vi "Douglas_22082017.vi"() -> ()   [LabVIEW 2017]
uses:
  <vilib>/Utility/error.llb/DialogType.ctl
  <vilib>/DAQmx/read.llb/DAQmx Read (Analog 1D Wfm NChan NSamp).vi
  <vilib>/Analysis/baseanly.llb/Mean (DBL).vi
  <vilib>/Analysis/5stat.llb/RMS (DBL).vi
  Instance           1 15Saved   Douglas .vi
  <vilib>/Waveform/WDTFileIO.llb/Export Waveforms To Spreadsheet File (1D).vi
  <vilib>/DAQmx/create/channels.llb/DAQmx Create Channel (AI-Voltage-Basic).vi
  <vilib>/DAQmx/configure/timing.llb/DAQmx Timing (Sample Clock).vi
  <vilib>/DAQmx/miscellaneous.llb/DAQmx Fill In Error Info.vi
  <vilib>/Waveform/WDTFileIO.llb/ Write Waveforms to File (1D).vi
  <vilib>/Analysis/NI_AALBase.lvlib
  <vilib>/Analysis/NI_AALPro.lvlib
panel:
  in  "Pasta":path=path "D:/Box Sync/Doctoring/Testes/DEF"
  in  "Nome do Arquivo":string="CTL_usado_BBA-CC-1,20_pre7"
  in  "Aquisição C/T":bool=TRUE
  in  "Aqusiçao de Temperatura":bool=TRUE
  in  "Tempo Temperatura [s]":i32=3
  out "Temperature":dynamicdata(graph)
  out "Potencia Media":dbl format="%0.2f"
  out "Current/Voltage":waveform(dbl)[](graph)
  out "Tensão RMS":dbl format="%0.2f"
  out "Tensão Média":dbl format="%0.2f"
  out "Corrente RMS":dbl format="%0.2f"
  out "Corrente Média":dbl format="%0.2f"
  in  "Taxa de Aquisição":dbl=6000.0 format="%0.2f"
  in  "Tempo de C/T [s]":i32=3
  in  "Canal":tag="Dev1/ai0:1"
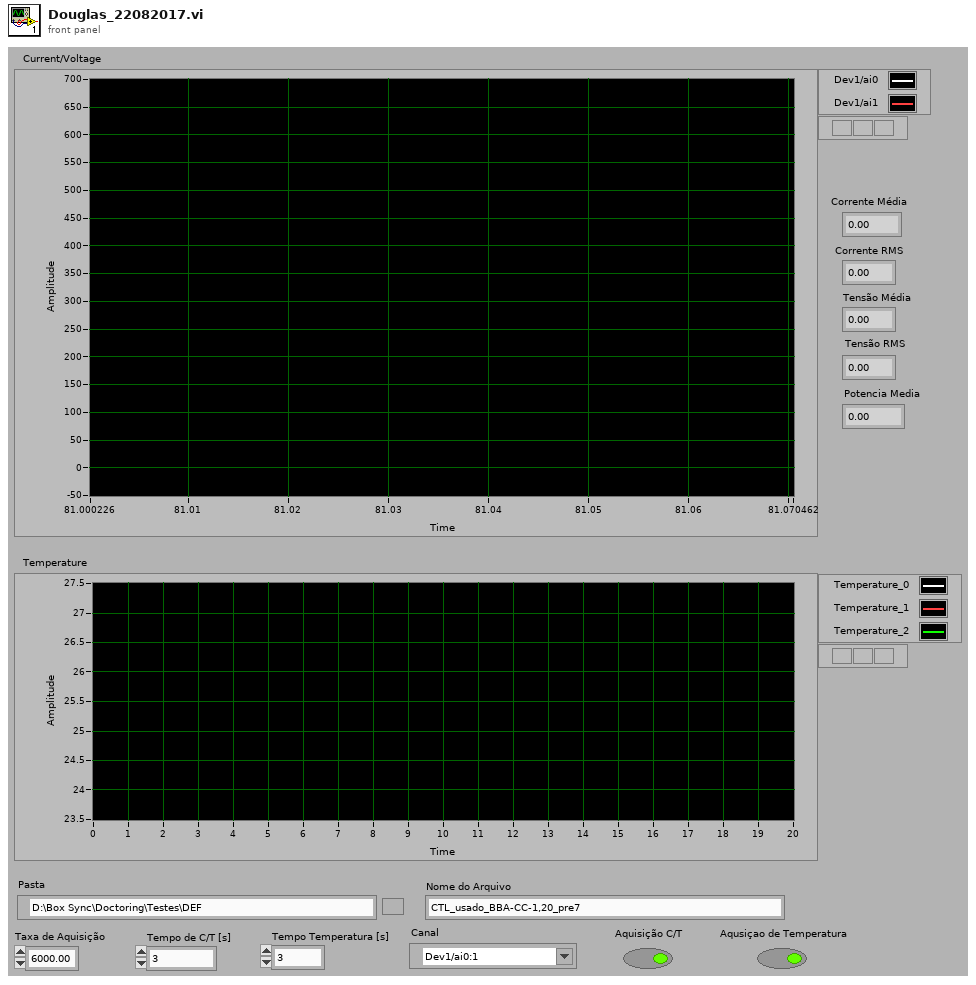
[diagram p1: front panel]
types:
  T1 = typedef "DialogType.ctl" = u16
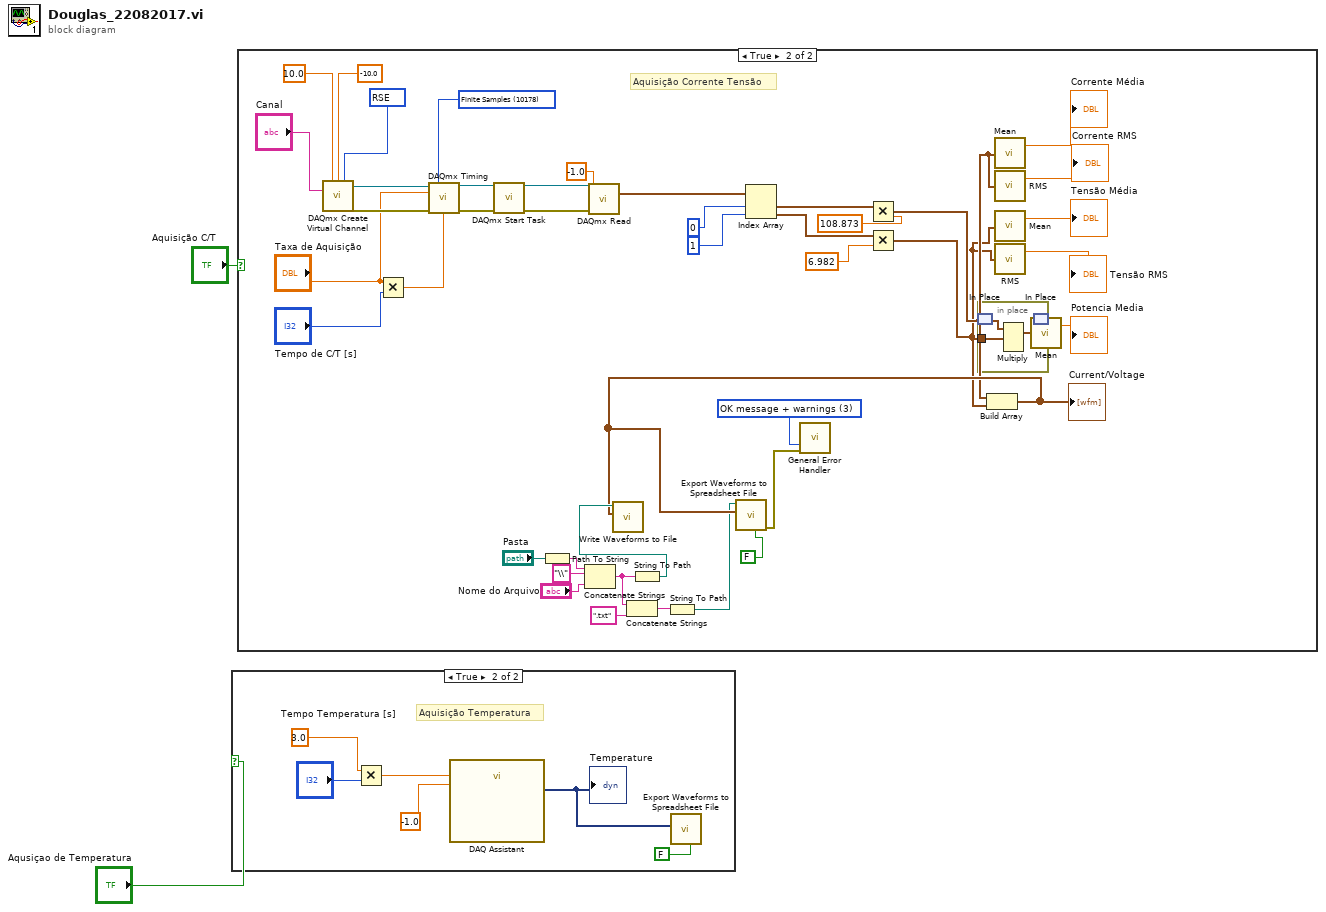
[diagram p0: block diagram]
diagram:
  n1 = case shown="True" "Aqusiçao de Temperatura" {
    frame False {
    }
    frame True {
      # "Aquisição Temperatura"
      n2 = Multiply(x=3.0 ("rate"), y="Tempo Temperatura [s]") -> (x*y=w7:dbl)
      n3 = call "DAQ Assistant"("number of samples"=w7, "timeout (s)"=-1.0) -> ("data"=w4:dynamicdata)  [unwired: 15 in, 2 out]
      "Temperature" <- w4
      n4 = call-poly <vilib>:"Export Waveforms to Spreadsheet File.vi"("header? (write header:T)"=FALSE, "waveforms"=w4) -> ()  [unwired: 8 in, 2 out]
    }
  }
  n5 = case shown="True" "Aquisição C/T" {
    frame False {
    }
    frame True {
      w13 = T1 3 items=["no dialog", "OK message", "continue or stop message", "OK message + warnings", "continue/stop + warnings"] ("type of dialog (OK msg:1)")
      w41 = 10178 items=["Finite Samples"=10178, "Continuous Samples"=10123, "Hardware Timed Single Point"=12522] ("sample mode")
      w42 = 10083 items=["default"=-1, "RSE"=10083, "NRSE"=10078, "Differential"=10106, "Pseudodifferential"=12529] ("input terminal configuration")
      # "Aquisição Corrente Tensão"
      n6 = call-poly <vilib>:"DAQmx Create Virtual Channel.vi"("maximum value"=10.0, "minimum value"=-10.0, "input terminal configuration"=w42, "physical channels"="Canal") -> ("task out"=w50:refnum<k21>, "error out"=w51:errorcluster)  [unwired: 10 in]
      n7 = Multiply(x="Taxa de Aquisição", y="Tempo de C/T [s]") -> (x*y=w28:dbl)
      n8 = call-poly <vilib>:"DAQmx Timing.vi"("task/channels in"=w50, "sample mode"=w41, "samples per channel"=w28, "rate"="Taxa de Aquisição", "error in"=w51) -> ("task out"=w49:refnum<k21>, "error out"=w48:errorcluster)  [unwired: 9 in]
      n9 = call <vilib>:"DAQmx Start Task.vi"("task/channels in"=w49, "error in"=w48) -> ("task out"=w47:refnum<k21>, "error out"=w46:errorcluster)  [unwired: 12 in]
      n10 = Path To String(path="Pasta") -> (string=w20:string)
      n11 = Concatenate Strings(w20, "\\" ("string"), "Nome do Arquivo") -> (w22:string)
      n12 = call-poly <vilib>:"DAQmx Read.vi"("task/channels in"=w47, "timeout"=-1.0, "error in"=w46) -> ("data"=w31:waveform(dbl)[])  [unwired: 10 in, 2 out]
      n13 = Concatenate Strings(w22, ".txt" ("string")) -> (w21:string)
      n14 = String To Path(string=w22) -> (path=w23:path)
      n15 = String To Path(string=w21) -> (path=w11:path)
      n16 = Index Array(array=w31, index #1=0 ("index"), index #2=1 ("index")) -> (element #1=w25:waveform(dbl), element #2=w26:waveform(dbl))
      n17 = Multiply(x=w25, y=108.873 ("x")) -> (x*y=w10:waveform(dbl))
      n18 = Multiply(x=w26, y=6.982) -> (x*y=w9:waveform(dbl))
      n19 = in-place {
        in-place-border: w9 -> [w53]
        n20 = in-place-match #1(w10) -> (w52:waveform(dbl))
        n21 = Multiply(1:w53, 2:w52) -> (0:w54:waveform(dbl))  [unwired: 1 in, 1 out]
        n22 = in-place-match #1(w54) -> (w29:waveform(dbl))
      }
      n23 = Build Array(w10, w9) -> (w12:waveform(dbl)[])
      "Current/Voltage" <- w12
      n24 = call-poly <vilib>:"Write Waveforms to File.vi"("waveform array"=w12, "file path (dialog if empty)"=w23) -> ()  [unwired: 8 in, 2 out]
      n25 = call-poly <vilib>:"Export Waveforms to Spreadsheet File.vi"("header? (write header:T)"=FALSE, "waveforms"=w12, "file path (dialog if empty)"=w11) -> ("error out"=w17:errorcluster)  [unwired: 7 in, 1 out]
      n26 = call <vilib>:"General Error Handler.vi"("type of dialog (OK msg:1)"=w13, "error in (no error)"=w17) -> ()  [unwired: 9 in, 5 out]
      n27 = call-poly <vilib>:"Mean.vi"("X"=w10) -> ("mean"=→"Corrente Média":dbl)  [unwired: 1 out]
      n28 = call-poly <vilib>:"RMS.vi"("X"=w10) -> ("rms value"=→"Corrente RMS":dbl)  [unwired: 1 out]
      n29 = call-poly <vilib>:"Mean.vi"("X"=w9) -> ("mean"=→"Tensão Média":dbl)  [unwired: 1 out]
      n30 = call-poly <vilib>:"RMS.vi"("X"=w9) -> ("rms value"=→"Tensão RMS":dbl)  [unwired: 1 out]
      n31 = call-poly <vilib>:"Mean.vi"("X"=w29) -> ("mean"=→"Potencia Media":dbl)  [unwired: 1 out]
    }
  }
